vi "OAT Full Spectrum (Orbit Plot).vi"(0 "orbit/timebase plot":T11(array[cluster]), 2 "window (Hanning)":T10=1 items=["None"=0, "Hanning"=1, "Hamming"=2, "Blackman-Harris"=3, "Exact Blackman"=4, "Blackman"=5, "Flat Top"=6, "4 Term B-Harris "=7, "7 Term B-Harris"=8, "Low Sidelobe"=9, "Force - Exponential"=10, "Force"=64, "Exponential"=65, "Blackman Nuttall"=11, "Triangle"=30, "Bartlett-Hanning"=31, "Bohman"=32, "Parzen"=33, "Welch"=34, "Kaiser"=60, "Dolph-Chebyshev"=61, "Gaussian"=62], 4 "view":T8={"dB On (F)"=FALSE, "unwrap phase (F)"=FALSE, "convert to degree (T)"=TRUE}, 5 "error in (no error)":errorcluster) -> (14 "full spectrum":T9, 15 "magnitude unit label":string, 16 "phase lag":T7 {"phase" format="%.2f"; "dOrder" format="%.2f"; "Order 0" format="%.2f"}, 17 "phase unit label":string, 18 "spectrum info":T1={"channel name"="", "description"="", "x-axis units"=0, "spectral info"={"spectrum type"=enum."Power [Magnitude^2]", "linear/dB"=enum."linear", "window"=0, "window size"=0, "FFT size"=0}, "engineering units"=0, "custom label"="", "dB reference [EU]"=0.0, "peak units"=enum."rms", "weighting filter"=0, "spectral density?"=FALSE, "unit label"="", "spectrum skewed?"=FALSE, "complimentary spectrum units"=enum."none"} {"x-axis units" items=["Time (s)"=0, "Frequency-CB (Hz)"=1, "Frequency-CPB (Hz)"=1248, "Frequency-Arbitrary (Hz)"=2357, "Quefrency (s)"=2, "Revolutions (rev)"=3, "Order"=4, "Speed (RPM)"=11, "Speed (rad/s)"=21, "Index"=65535]; "weighting filter" items=["Linear", "A-weighting", "B-weighting", "C-weighting", "ITU-R 468-4", "Dolby", "CCITT", "C-message", "Wb", "Wc", "Wd", "We", "Wf", "Wh", "Wj", "Wk", "Wm", "AES17 20 kHz lowpass", "AES17 40 kHz lowpass", "AES17 20 kHz highpass", "AES17 40 kHz highpass"]; "dB reference [EU]" format="%.2f"; "engineering units" items=["custom..."=0, "V"=1, "A"=21, "C"=30, "pC"=31, "s"=32, "-"=29, "Pa"=2, "N"=20, "g"=3, "m/s^2"=4, "m/s"=5, "m"=6, "mm/s"=12, "mm"=13, "micron/s"=14, "micron"=15, "in/s^2"=7, "in/s"=8, "in"=9, "mil/s"=10, "mil"=11, "rad/s^2"=16, "rad/s"=17, "rad"=18, "deg/s^2"=26, "deg/s"=27, "deg"=28, "RPM"=22, "cycle/s^2"=23, "Hz"=24, "cycle"=25, "strain"=19]; "spectral info"."window" items=["None "=0, "Hanning"=1, "Hamming"=2, "Blackman-Harris"=3, "Exact Blackman"=4, "Blackman"=5, "Flat Top"=6, "4 Term B-Harris "=7, "7 Term B-Harris"=8, "Low Sidelobe"=9, "Force - Exponential"=10, "Gaussian"=62]}, 19 "error out":errorcluster)   [LabVIEW 2017, in "SoundVib_OrderTracking.lvlib"]
doc: "This VI computes the full spectrum of a probe pair. The full spectrum provides information on the amplitude of vibration as well as the orbit eccentricity and direction of precession for each frequency/order component."
uses:
  <vilib>/addons/Sound and Vibration/Order Analysis/Resample Order Tracking/SoundVib_OrderTracking.lvlib
  <vilib>/addons/_NISVFA/_Shared subVIs/Controls/svc_Window [Dual FFT].ctl
  <vilib>/addons/_NISVFA/_Shared subVIs/Controls/svc_Spectrum Info.ctl
  <vilib>/addons/_NISVFA/_Shared subVIs/Controls/svc_X-Axis Units.ctl
  <vilib>/addons/_NISVFA/_Shared subVIs/Controls/svc_Spectrum Type.ctl
  <vilib>/addons/_NISVFA/_Shared subVIs/Controls/svc_Engineering Units Text Ring.ctl
  <vilib>/addons/_NISVFA/_Shared subVIs/Controls/svc_Weighting Filter Text Ring.ctl
  <vilib>/addons/_NISVFA/_Shared subVIs/Controls/svc_Complimentary Spectrum Units.ctl
  <vilib>/addons/_NISVFA/_Shared subVIs/Controls/svc_Resampled Channel Info.ctl
  <vilib>/addons/_NISVFA/_Shared subVIs/Controls/svc_Channel Info.ctl
  <vilib>/addons/Sound and Vibration/Order Analysis/Misc/SVMS Attribute.ctl
  <vilib>/addons/_NISVFA/_Shared subVIs/Controls/NI Channel Properties.ctl
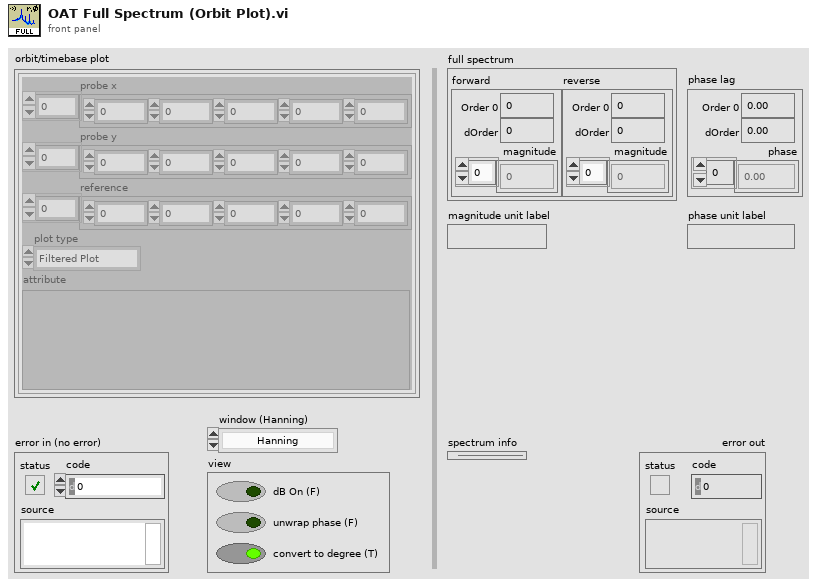
[diagram p1: front panel]
types:
  T1 = typedef "svc_Spectrum Info.ctl" = cluster{"channel name":string, "description":string, "x-axis units":T2, "spectral info":cluster{"spectrum type":T3, "linear/dB":enum16{"linear", "dB"}, "window":u16, "window size":i32, "FFT size":i32}, "engineering units":T4, "custom label":string, "dB reference [EU]":dbl, "peak units":enum16{"rms", "peak", "peak-peak"}, "weighting filter":T5, "spectral density?":bool, "unit label":string, "spectrum skewed?":bool, "complimentary spectrum units":T6}
  T2 = typedef "svc_X-Axis Units.ctl" = u16
  T3 = typedef "svc_Spectrum Type.ctl" = enum16{"FFT Spectrum [complex]", "Amplitude [Magnitude]", "Power [Magnitude^2]", "Cross Spectrum [complex]", "Frequency Response [Complex]"}
  T4 = typedef "svc_Engineering Units Text Ring.ctl" = u16
  T5 = typedef "svc_Weighting Filter Text Ring.ctl" = u16
  T6 = typedef "svc_Complimentary Spectrum Units.ctl" = enum16{"none", "radians", "degrees", "cycles", "imaginary"}
  T7 = cluster{"Order 0":dbl, "dOrder":dbl, "phase":dbl[]}
  T8 = cluster{"dB On (F)":bool, "unwrap phase (F)":bool, "convert to degree (T)":bool}
  T9 = cluster{"forward":cluster{"Order 0":dbl, "dOrder":dbl, "magnitude":dbl[]}, "reverse":cluster{"Order 0":dbl, "dOrder":dbl, "magnitude":dbl[]}}
  T10 = typedef "svc_Window [Dual FFT].ctl" = u32
  T11 = cluster{"probe x":dbl[], "probe y":dbl[], "reference":dbl[], "plot type":enum16{"Filtered Plot", "Unfiltered Plot"}, "attribute":variant}[][]
  T12 = typedef "svc_Resampled Channel Info.ctl" = cluster{"channel name":string, "description":string, " channel info":T13}
  T13 = typedef "svc_Channel Info.ctl" = cluster{"sensor sensitivity":dbl, "engineering units":T4, "dB reference":dbl, "custom label":string, "weighting filter":T5, "pregain":dbl}
  T14 = typedef "NI Channel Properties.ctl" = u16
  T15 = typedef "SVMS Attribute.ctl" = u16
  T16 = cluster{"probe x":dbl[], "probe y":dbl[], "reference":dbl[], "plot type":enum16{"Filtered Plot", "Unfiltered Plot"}, "attribute":variant}
  T17 = cluster{"averaging mode":enum16{"No averaging", "Vector averaging", "RMS averaging", "Peak hold"}, "weighting mode":enum16{"Linear", "Exponential"}, "number of averages":u32, "linear mode":enum16{"One shot", "Auto restart"}}
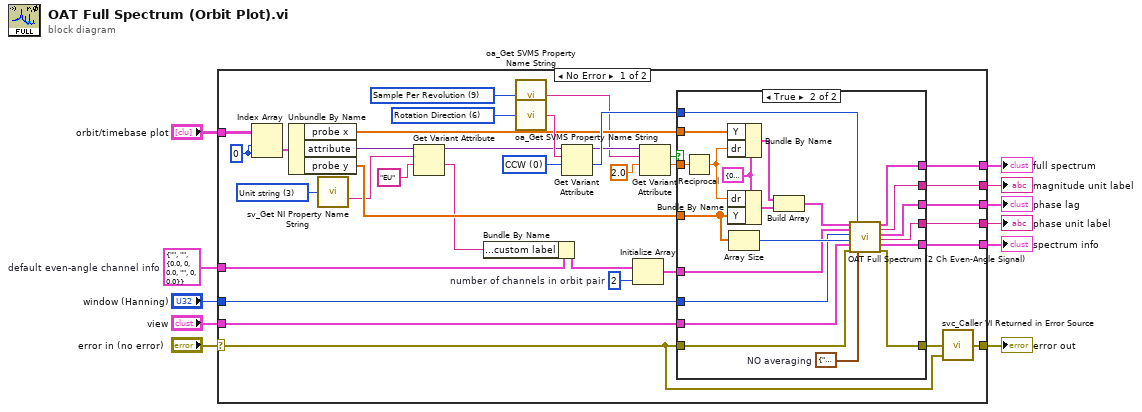
[diagram p0: block diagram]
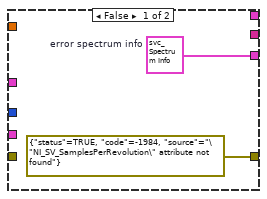
[diagram p2: hidden frame]
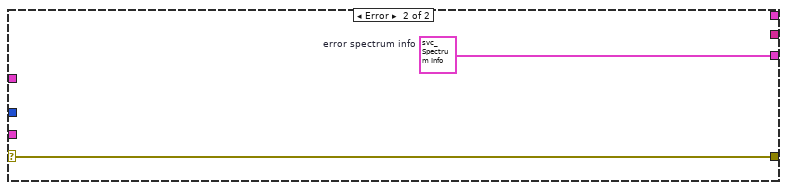
[diagram p3: hidden frame]
diagram:
  w1 = T12 {"channel name"="", "description"="", " channel info"={"sensor sensitivity"=0.0, "engineering units"=0, "dB reference"=0.0, "custom label"="", "weighting filter"=0, "pregain"=0.0}}  # default even-angle channel info
  n1 = case shown="No Error" "error in (no error)" {
    selector: "error in (no error)" -> [w28 w71]
    tunnel: [w27 _] -> w11
    tunnel: "orbit/timebase plot" -> [w30 _]
    tunnel: "view" -> [w29 _]
    tunnel: [w46 w71] -> w8
    tunnel: [w25 _] -> w7
    tunnel: [w26 w70] -> w6
    tunnel: "window (Hanning)" -> [w31 _]
    tunnel: [w21 _] -> w3
    tunnel: [w20 _] -> w2
    tunnel: w1 -> [w18 _]
    frame No Error {
      w19 = T14 3 items=["Channel name", "Channel description", "Axis label", "Unit string", "Waveform X-axis label", "Waveform X-axis unit string", "x0", "dx", "Number of samples", "X channel", "Filter settled", "dB reference", "Window", "Window parameter", "Window size", "FFT size", "Peak units", "Spectrum type", "Magnitude scale", "Spectral density", "Sensor sensitivity (mV/EU)", "X-axis dimension", "LabVIEW datatype", "Function type", "Function subtype", "X values", "Independent channel", "Column index", "Collection name", "Collection ID", "X Columns", "Phase unwrapped", "Sensor type", "Sensor maximum", "Averaging mode"] ("property")
      w44 = 2  # number of channels in orbit pair
      w42 = u16 0 items=["CCW", "CW"] ("direction")
      w36 = 0 ("disabled index (col)")
      w33 = T15 9 items=["Pulse / Revolution", "Slope", "Threshold", "Hysteresis", "Order", "Reference Label", "Rotation Direction", "Pair String", "Polar Plot Type", "Sample Per Revolution", "Probe Angle", "Probe Angle X", "Probe Angle Y", "X Axis Unit", "OTB Plot Type"] ("attribute")
      w32 = T15 6 items=["Pulse / Revolution", "Slope", "Threshold", "Hysteresis", "Order", "Reference Label", "Rotation Direction", "Pair String", "Polar Plot Type", "Sample Per Revolution", "Probe Angle", "Probe Angle X", "Probe Angle Y", "X Axis Unit", "OTB Plot Type"] ("attribute")
      n2 = Index Array(array=w30, index (row)=w36, index (col)=w36) -> (element=w34:T16)
      n3 = Unbundle By Name(w34) -> ("probe x"=w39:dbl[], "attribute"=w15:variant, "probe y"=w23:dbl[])
      n4 = call <vilib>:"sv_Get NI Property Name String.vi"("property"=w19) -> ("WDT attribute name"=w14:string)  [unwired: 13 in, 1 out]
      n5 = Get Variant Attribute(Variant=w15, name=w14, default value (empty Variant)="EU" ("WDT attribute name")) -> (duplicate Variant=w16:variant, value=w12:string)  [unwired: 1 in, 2 out]
      n6 = Bundle By Name(cluster=w18, "channel info.custom label"=w12) -> (w17:T12)
      n7 = call <vilib>:"oa_Get SVMS Property Name String.vi"("attribute"=w33) -> ("attribute name"=w35:string)  [unwired: 4 in]
      n8 = call <vilib>:"oa_Get SVMS Property Name String.vi"("attribute"=w32) -> ("attribute name"=w41:string)  [unwired: 4 in]
      n9 = Get Variant Attribute(Variant=w16, name=w41, default value (empty Variant)=w42) -> (duplicate Variant=w40:variant, value=w43:u16)  [unwired: 1 in, 2 out]
      n10 = Initialize Array(w17, w44) -> (w45:T12[])
      n11 = Get Variant Attribute(Variant=w40, name=w35, default value (empty Variant)=2.0 ("max order (auto)")) -> (found=w22:bool, value=w38:dbl)  [unwired: 1 in, 2 out]
      n12 = case shown="True" w22 {
        tunnel: w45 -> [_ w68]
        tunnel: w43 -> [_ w67]
        tunnel: w39 -> [_ w63]
        tunnel: w38 -> [_ w61]
        tunnel: w31 -> [_ w60]
        tunnel: w29 -> [_ w59]
        tunnel: w28 -> [_ w57]
        tunnel: [_ w56] -> w27
        tunnel: [w48 w55] -> w26
        tunnel: [_ w54] -> w25
        tunnel: [errorcluster {"status"=TRUE, "code"=-1984, "source"="\"NI_SV_SamplesPerRevolution\" attribute not found"} ("error out") w53] -> w24
        tunnel: w23 -> [_ w51]
        tunnel: [_ w50] -> w21
        tunnel: [_ w49] -> w20
        frame False {
          w48 = T1 {"channel name"="Error", "description"="Error", "x-axis units"=99, "spectral info"={"spectrum type"=enum."Power [Magnitude^2]", "linear/dB"=enum."linear", "window"=99, "window size"=-1, "FFT size"=-1}, "engineering units"=0, "custom label"="Error", "dB reference [EU]"=0.0, "peak units"=enum."rms", "weighting filter"=0, "spectral density?"=FALSE, "unit label"="Error", "spectrum skewed?"=FALSE, "complimentary spectrum units"=enum."none"}  # error spectrum info
        }
        frame True {
          w58 = T17 {"averaging mode"=enum."No averaging", "weighting mode"=enum."Exponential", "number of averages"=10, "linear mode"=enum."One shot"}  # NO averaging
          w62 = cluster{"r0":dbl, "dr":dbl, "Y":dbl[]} {"r0"=0.0, "dr"=1.0, "Y"=[]} ("even angle signal")
          n13 = Reciprocal(x=w61) -> (1/x=w52:dbl)
          n14 = Bundle By Name(cluster=w62, "Y"=w63, "dr"=w52) -> (w64:cluster{"r0":dbl, "dr":dbl, "Y":dbl[]})
          n15 = Bundle By Name(cluster=w62, "dr"=w52, "Y"=w51) -> (w65:cluster{"r0":dbl, "dr":dbl, "Y":dbl[]})
          n16 = Array Size(array=w51) -> (size(s)=w69:i32)
          n17 = Build Array(w64, w65) -> (w66:cluster{"r0":dbl, "dr":dbl, "Y":dbl[]}[])
          n18 = call <vilib>:"OAT Full Spectrum (2 Ch Even-Angle Signal).vi"("even-angle signals"=w66, "even-angle channel info"=w68, "window (Hanning)"=w60, "block size (-1 = automatic)"=w69, "view"=w59, "error in (no error)"=w57, "rotation direction (CCW)"=w67, "averaging parameters"=w58) -> ("full spectrum"=w56:T9, "magnitude unit label"=w49:string, "phase lag"=w54:T7, "phase unit label"=w50:string, "spectrum info"=w55:T1, "error out"=w53:errorcluster)  [unwired: 3 in, 3 out]
        }
      }
      n19 = call <vilib>:"svc_Caller VI Returned in Error Source.vi"("warning input to caller"=w28, "error in (no error)"=w24) -> ("error out"=w46:errorcluster)  [unwired: 3 in]
    }
    frame Error {
      w70 = T1 {"channel name"="Error", "description"="Error", "x-axis units"=99, "spectral info"={"spectrum type"=enum."Power [Magnitude^2]", "linear/dB"=enum."linear", "window"=99, "window size"=-1, "FFT size"=-1}, "engineering units"=0, "custom label"="Error", "dB reference [EU]"=0.0, "peak units"=enum."rms", "weighting filter"=0, "spectral density?"=FALSE, "unit label"="Error", "spectrum skewed?"=FALSE, "complimentary spectrum units"=enum."none"}  # error spectrum info
    }
  }
  "full spectrum" <- w11
  "phase lag" <- w7
  "error out" <- w8
  "spectrum info" <- w6
  "phase unit label" <- w3
  "magnitude unit label" <- w2
